vi "tm_opendcimgfile.vi"(8 "error in (no error)":errorcluster, 11 "Path":path) -> (0 "error out":errorcluster, 2 "Total Frames":i32, 3 "File Handle":u32)   [LabVIEW 2015]
uses:
  tmcamcon.dll
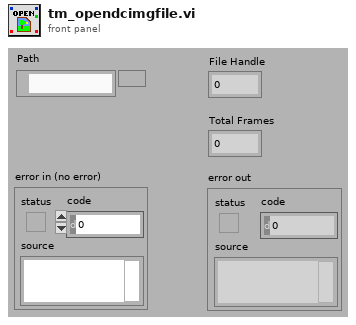
[diagram p1: front panel]
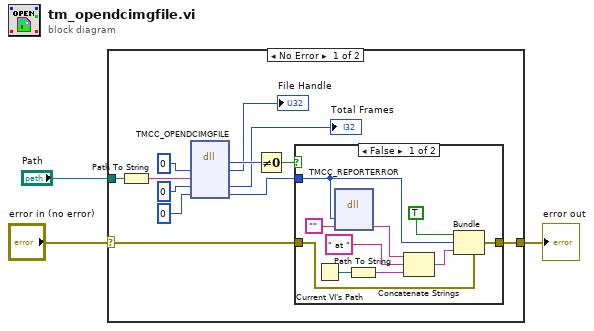
[diagram p0: block diagram]
diagram:
  n1 = case shown="No Error" "error in (no error)" {
    selector: "error in (no error)" -> [w11 w27]
    tunnel: [w10 w27] -> w2
    tunnel: "Path" -> [w5 _]
    frame No Error {
      n2 = Path To String(path=w5) -> (string=w4:string)
      n3 = dll-call lib="tmcamcon.dll" fn="TMCC_OPENDCIMGFILE"("filehandle"=u32 0, "path"=w4, "totalframes"=0, "Erval"=0) -> ("return type"=w15:u32, "filehandle"=→"File Handle":u32, "totalframes"=→"Total Frames":i32, "Erval"=w13:i32)  [unwired: 4 in, 2 out]
      n4 = Not Equal To 0?(x=w15) -> (x != 0?=w12:bool)
      n5 = case shown="False" w12 {
        tunnel: w11 -> [w25 w26]
        tunnel: [w24 w26] -> w10
        tunnel: w13 -> [w18 _]
        frame False {
          n6 = Current VI's Path() -> (path=w23:path)
          n7 = dll-call lib="tmcamcon.dll" fn="TMCC_REPORTERROR"("error"=w18, "buf"="") -> ("buf"=w17:string)  [unwired: 5 in, 2 out]
          n8 = Path To String(path=w23) -> (string=w19:string)
          n9 = Concatenate Strings(w17, " at ", w19) -> (w22:string)
          n10 = Bundle(cluster=w25, "status"=TRUE, "code"=w18, "source"=w22) -> (w24:errorcluster)
        }
        frame True {
        }
      }
    }
    frame Error {
    }
  }
  "error out" <- w2
